vi "file_pha app.vi"() -> ()   [LabVIEW 2012, in "LightPipes.lvlib"]
uses:
  LightPipes.lvlib
panel:
  out "field out":T1={"n_grid"=256, "@dummy control@"=0, "@dummy control@"=0, "@dummy control@"=0, "@dummy control@"=0, "size"=0.01, "lambda"=1e-06, "int1"=0, "int2"=0, "int3"=0, "@dummy control@"=0, "@dummy control@"=0, "@dummy control@"=0, "@dummy control@"=0, "double1"=0.0, "double2"=0.0, "double3"=0.0, "real"=296878144, "imaginary"=297467968}
  # "Images"
  # "PHASE PRINTING"
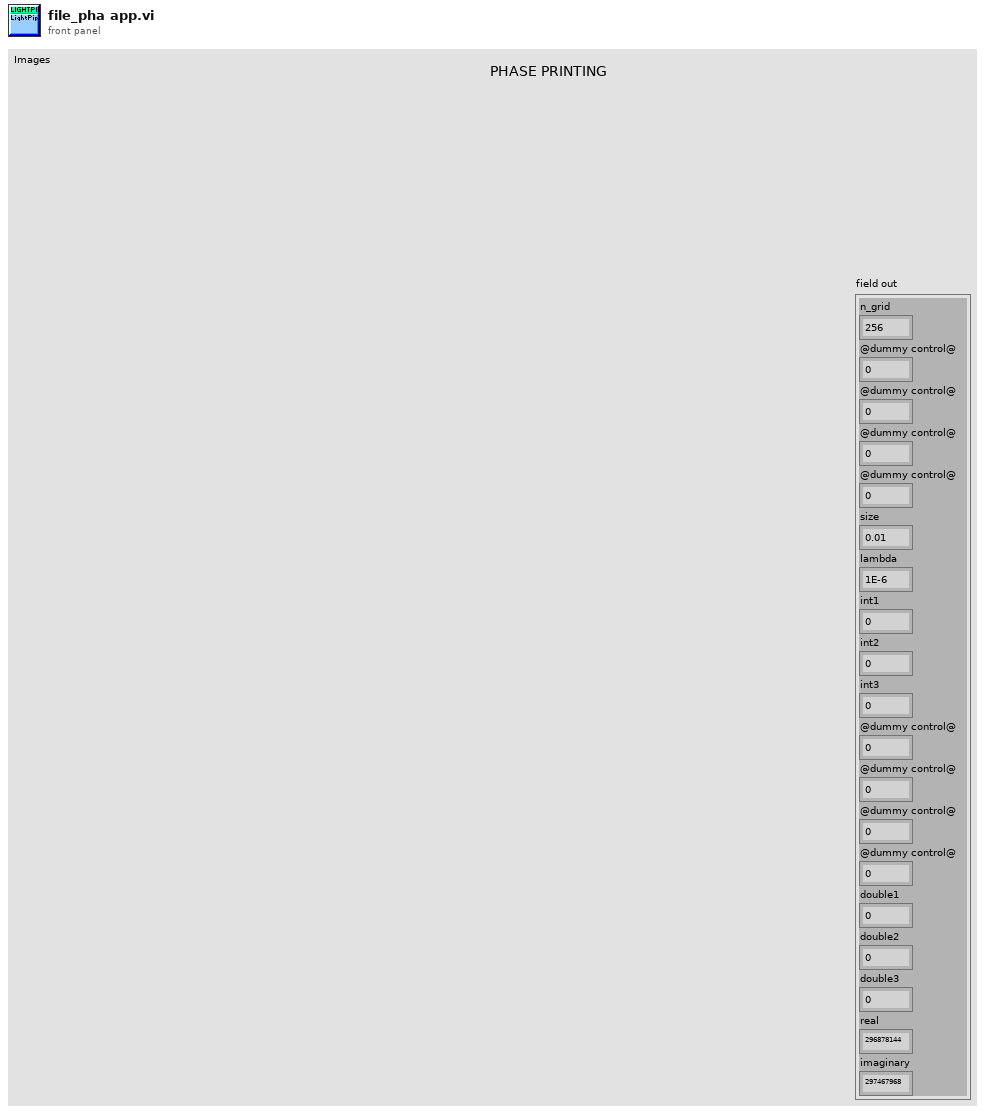
[diagram p1: front panel]
types:
  T1 = cluster{"n_grid":i32, "@dummy control@":i8, "@dummy control@":i8, "@dummy control@":i8, "@dummy control@":i8, "size":dbl, "lambda":dbl, "int1":i32, "int2":i32, "int3":i32, "@dummy control@":i8, "@dummy control@":i8, "@dummy control@":i8, "@dummy control@":i8, "double1":dbl, "double2":dbl, "double3":dbl, "real":u32, "imaginary":u32}
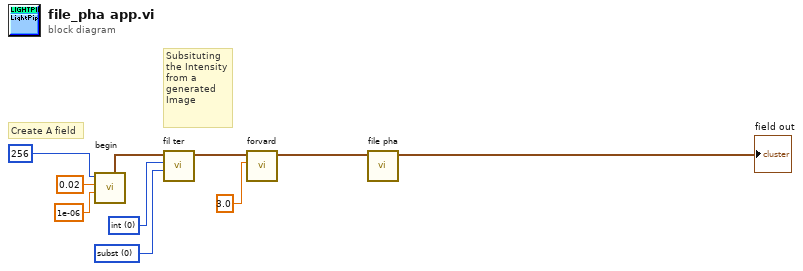
[diagram p0: block diagram]
diagram:
  w7 = i16 0 items=["int", "pha"] ("intensity / phase")
  w6 = i16 0 items=["subst", "mult"] ("multiplication/ substitution")
  # "Create A field"
  # "Subsituting the Intensity from a generated Image"
  n1 = call "begin.vi"("lambda"=1e-06, "size_grid"=0.02, "n_grid"=256) -> ("field out"=w5:T1)  [unwired: 8 in]
  n2 = call "fil ter.vi"("multiplication/ substitution"=w6, "intensity / phase"=w7, "field"=w5) -> ("field out"=w3:T1)  [unwired: 7 in, 1 out]
  n3 = call "forvard.vi"("distance"=3.0, "field"=w3) -> ("field out"=w4:T1)  [unwired: 9 in]
  n4 = call "file pha.vi"("field"=w4) -> ("field out"=→"field out":T1)  [unwired: 9 in, 1 out]
